vi "Recipe array ausgeben.vi"(0 "Komplette Datei":string, 11 "error in (no error)":errorcluster caption="Fehler (Eingang, kein Fehler)") -> (4 "Recipe Teil":string[][](array[string]), 6 "Rezpt nicht gefunden":bool, 8 "END nicht gefunden":bool, 15 "error out":errorcluster caption="Fehler (Ausgang)")   [LabVIEW 2020, in "AK-Schnittstelle.lvlib"]
uses:
  AK-Schnittstelle.lvlib
  Stoerungen/Stoerungen Messgeraet/Aktionen Kommunikation Stoerung.ctl
  Seiten/FT-IR/FGV FT-IR Aktionen.ctl
  Stoerungen/Stoerungen.lvlib
  Seiten/FT-IR/FT-IR.lvlib
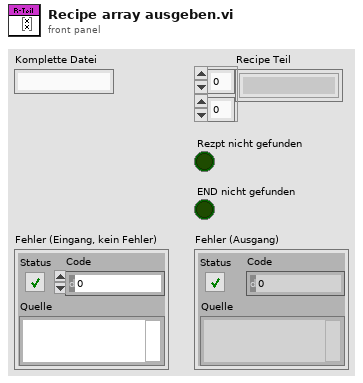
[diagram p1: front panel]
types:
  T1 = typedef "FT-IR.lvlib/FGV FT-IR Aktionen.ctl" = enum16{"lesen", "NOG setzen", "NOS setzen", "Initialisieren", "speichern", "ALLES setzen", "FT-IR Spektrum loggen", "Komm Stoppen", "Spektrum LogKonfig"}
  T2 = typedef "Stoerungen.lvlib/Aktionen Kommunikation Stoerung.ctl" = enum16{"lesen", "init", "FT-IR Komm", "FT-IR Betriebsart", "FT-IR Hintergrund", "cRIO Komm", "PNS Komm", "Dichtheitstest", "Life Bit", "FTIR Komm AK", "PMA Komm", "FID Komm", "PMA Cal", "FID Ch4 Cal", "FID THC Cal", "Cal Timeout", "VFS 1 Komm", "VFS 2 Komm", "VFS 3 Komm", "VFS 4 Komm", "TRE 08 Komm", "CG-Test vorzeitig", "CG-Test Span 1", "CG-Test Span 2", "CG-Test Span 3", "CG-Test Messgas", "CG-Test löschen", "Test", "Amium AK", "AK Recept konfig", "AK Name konfig", "AK EKFG konfig"}
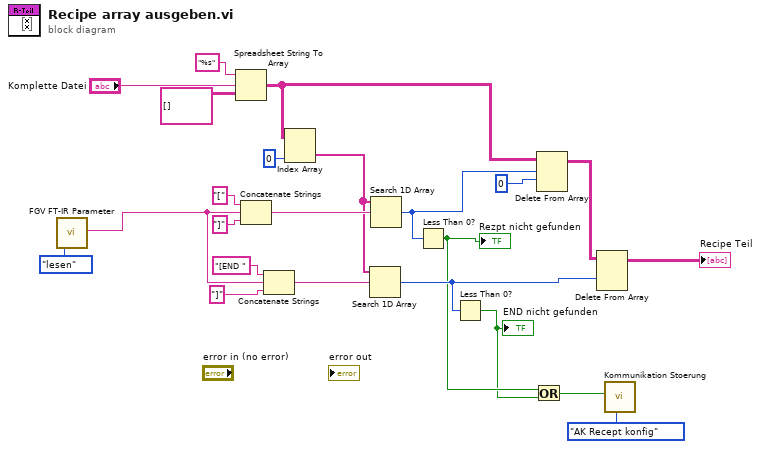
[diagram p0: block diagram]
diagram:
  n1 = call "FGV FT-IR Parameter.vi"("Aktion"=FGV_FT-IR_Aktionen."lesen") -> ("Current Recipe"=w1:string)  [unwired: 11 in, 7 out]
  n2 = Spreadsheet String To Array(format string="%s" ("Format-String"), spreadsheet string="Komplette Datei", array type (2D Dbl)=string[][] []) -> (array=w11:string[][])  [unwired: 1 in]
  n3 = Concatenate Strings("[" ("String"), w1, "]" ("String")) -> (w19:string)
  n4 = Concatenate Strings("[END " ("String"), w1, "]" ("String")) -> (w18:string)
  n5 = Index Array(array=w11, index (col)=0 ("Deaktivierter Index (Spalte)")) -> (element=w10:string[])  [unwired: 1 in]
  n6 = Search 1D Array(1D array=w10, element=w18) -> (index of element=w7:i32)  [unwired: 1 in]
  n7 = Search 1D Array(1D array=w10, element=w19) -> (index of element=w8:i32)  [unwired: 1 in]
  n8 = Less Than 0?(x=w8) -> (x < 0?=w4:bool)
  "Rezpt nicht gefunden" <- w4
  n9 = Less Than 0?(x=w7) -> (x < 0?=w3:bool)
  "END nicht gefunden" <- w3
  n10 = Or(x=w4, y=w3) -> (x .or. y?=w5:bool)
  n11 = Delete From Array(array=w11, length=w8, index (row)=0 ("Index (Zeile)")) -> (array with subset deleted=w13:string[][])  [unwired: 1 in, 1 out]
  n12 = Delete From Array(array=w13, index (row)=w7) -> (array with subset deleted=→"Recipe Teil":string[][])  [unwired: 2 in, 1 out]
  n13 = call "Kommunikation Stoerung.vi"("Aktionen"=Aktionen_Kommunikation_Stoerung."AK Recept konfig", "ERROR"=w5) -> ()  [unwired: 9 in, 1 out]
